vi "Create Project Report.vi"() -> ()   [LabVIEW 2013]
doc: "This example illustrates how to create a test report for all tests in a project."
uses:
  <vilib>/addons/_JKI Toolkits/Caraya/classes/Test Runner.Project/Test Runner.Project.lvclass
  JUnit for Azure Pipelines/JUnit for Azure Pipelines.lvclass
  <vilib>/addons/_JKI Toolkits/Caraya/classes/Test Runner/Test Runner.lvclass
panel:
  out "error out":errorcluster
  in  "Path":path
  # "1) Specify a path to store the test report file.\n2) Run the VI and review the created file.\n\nSee the block diagram for more information."
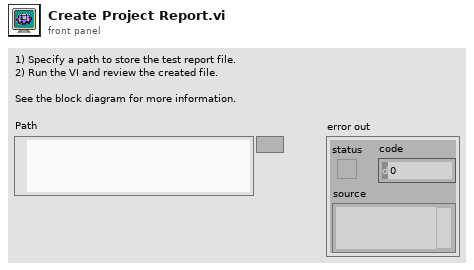
[diagram p1: front panel]
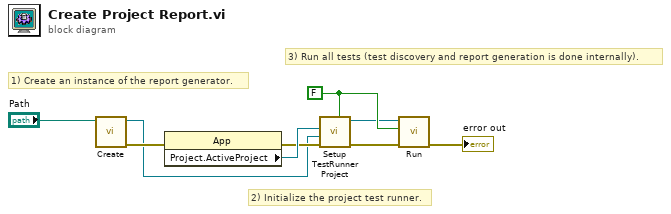
[diagram p0: block diagram]
diagram:
  w3 = FALSE ("Interactive (T)")
  # "3) Run all tests (test discovery and report generation is done internally)."
  # "2) Initialize the project test runner."
  # "1) Create an instance of the report generator."
  n1 = call "Create.vi"("Path"="Path") -> ("error out"=w7:errorcluster, "JUnit for Azure Pipelines"=w5:refnum<class "JUnit for Azure Pipelines.lvclass">)  [unwired: 9 in]
  n2 = property class="App"(error in=w7) -> (error out=w6:errorcluster, "Project.ActiveProject"=w9:refnum<vi>)  [unwired: 1 in, 1 out]
  n3 = call <vilib>:"Setup TestRunner Project.vi"("Interactive (T)"=w3, "error in (no error)"=w6, "Test Report"=w5, "Project Refnum"=w9) -> ("error out"=w4:errorcluster, "Test Runner.Project out"=w1:refnum<class "Test Runner.Project.lvclass">)  [unwired: 6 in]
  n4 = call <vilib>:"Run.vi"("error in (no error)"=w4, "Interactive"=w3, "Test Runner in"=w1) -> ("error out"=→"error out":errorcluster)  [unwired: 6 in, 2 out]
